vi "Check_and_edit_Scan_table.vi"(3 "2D array input":dbl[][](array[numeric]) format="%.2f", 4 "Original Channels":string[](array[string]), 5 "Present Channels":string[](array[string])) -> (0 "2D array output":dbl[][](array[numeric]) format="%.2f", 2 "Merged?":bool)   [LabVIEW 2010]
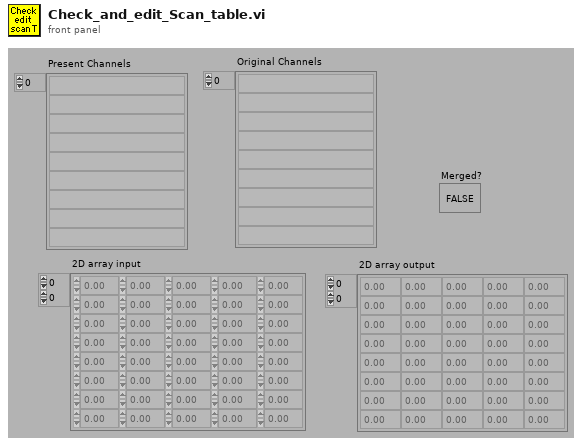
[diagram p1: front panel]
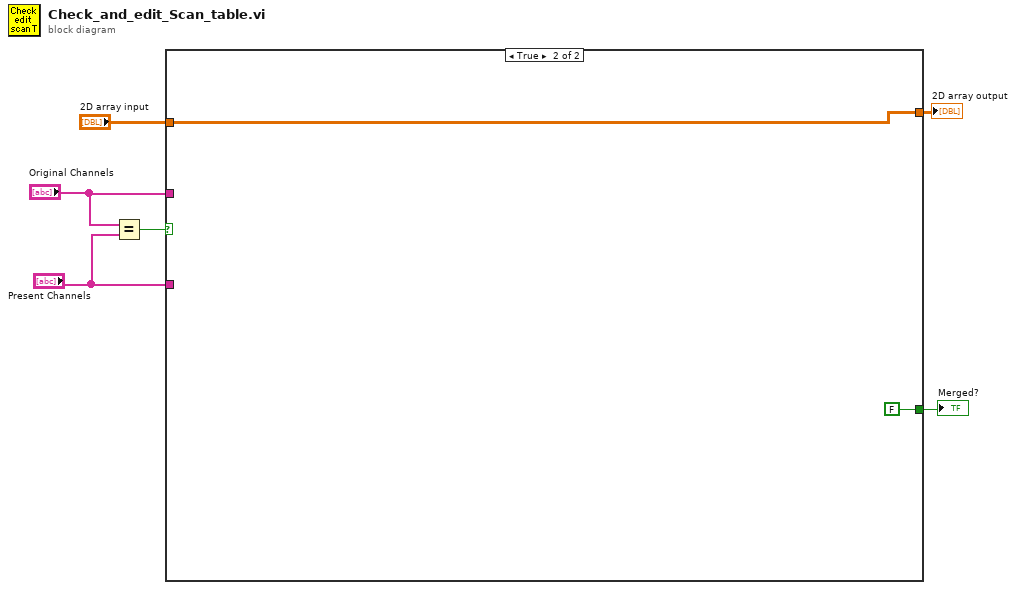
[diagram p0: block diagram]
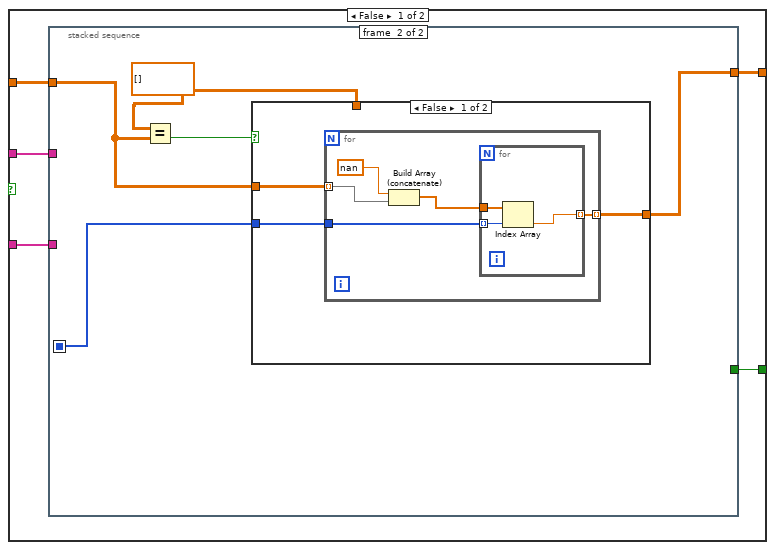
[diagram p2: hidden frame]
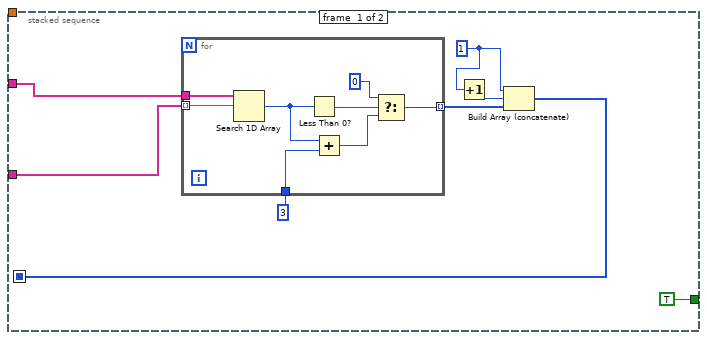
[diagram p3: hidden frame]
diagram:
  n1 = Equal?(x="Original Channels", y="Present Channels") -> (x = y?=w4:bool)
  n2 = case shown="True" w4 {
    tunnel: [w11 FALSE] -> w3
    tunnel: "Present Channels" -> [w10 _]
    tunnel: "Original Channels" -> [w9 _]
    tunnel: "2D array input" -> [w8 w45]
    tunnel: [w7 w45] -> w1
    frame False {
      n3 = stacked-sequence {
        seq-local: [w14 _] -> [_ w32]
        tunnel: [TRUE _] -> w11
        tunnel: w10 -> [w19 _]
        tunnel: w9 -> [w18 _]
        tunnel: w8 -> [_ w30]
        tunnel: [_ w31] -> w7
        frame #0 {
          w13 = 1 ("t")
          n4 = for {
            tunnel: [w25] -> w15 mode=indexing
            tunnel: w19 -> [w24] mode=indexing
            tunnel: w18 -> [w23]
            tunnel: 3 ("y") -> [w20]
            n5 = Search 1D Array(1D array=w23, element=w24) -> (index of element=w22:i32)  [unwired: 1 out]
            n6 = Less Than 0?(x=w22) -> (x < 0?=w27:bool)
            n7 = Add(x=w22, y=w20) -> (x+y=w21:i32)
            n8 = Select(t=0, s=w27, f=w21) -> (s? t:f=w25:i32)
          }
          n9 = Increment(x=w13) -> (x+1=w12:i32)
          n10 = Build Array (concatenate)(w13, w12, w15) -> (w14:i32[])
        }
        frame #1 {
          w28 = dbl[][] [] ("2D array input")
          n11 = Equal?(x=w28, y=w30) -> (x = y?=w29:bool)
          n12 = case shown="False" w29 {
            tunnel: w32 -> [w35 _]
            tunnel: [w34 w44] -> w31
            tunnel: w30 -> [w33 _]
            tunnel: w28 -> [_ w44]
            frame False {
              n13 = for {
                tunnel: w33 -> [w39] mode=indexing
                tunnel: w35 -> [w40]
                tunnel: [w36] -> w34 mode=indexing
                n14 = Build Array (concatenate)(nan, w39) -> (w38:dbl[])
                n15 = for {
                  tunnel: w38 -> [w43]
                  tunnel: w40 -> [w42] mode=indexing
                  tunnel: [w41] -> w36 mode=indexing
                  n16 = Index Array(array=w43, index=w42) -> (element=w41:dbl)
                }
              }
            }
            frame True {
            }
          }
        }
      }
    }
    frame True {
    }
  }
  "Merged?" <- w3
  "2D array output" <- w1
